vi "DAQ Thread_Gantner.vi"() -> ()   [LabVIEW 2016]
uses:
  HardWare/Gantner/HW_DevInfo.ctl
  HardWare/Gantner/HW_Module Info.ctl
  HardWare/Ctrls/HardWare Basic Info _ Channel.ctl
  HardWare/Ctrls/HardWare _ Channel Parameters.ctl
  Ctrls/Read and Write Ring.ctl
  HardWare/Gantner/DAQ FGV Operations.ctl
  Architecture/Queue Management/ARC_Queue Create_Single.vi
  Architecture/Queue Management/ARC_Queue Valid.vi
  Architecture/Queue Management/ARC_Queue Remove Element.vi
  Architecture/Queue Management/ARC_Queue Insert Element.vi
  Architecture/Queue Management/ARC_Queue Destroy_Single.vi
  <vilib>/Utility/error.llb/DialogType.ctl
panel:
  in  "daq?":bool
  in  "Parameter":cluster{"Q-Local":string, "Variant":variant}
  out "Error Report":string
  out "Current State":string
  in  "Exit Program":bool
  in  "TempVariable":T5
  # "/* -------- Notes for All Users -------- */\nRecommand : \n[1].Display Setting Resolution -> 1440x900\n[2].Read Arch Notes First.\n[3].Make A Call When You Are In Trouble.\n\nTeam Members:\nPansino Soft,Pansino SDMA\n\nCopyright@2013 Pansino.Beijing\n\nVersion Number: 2013"
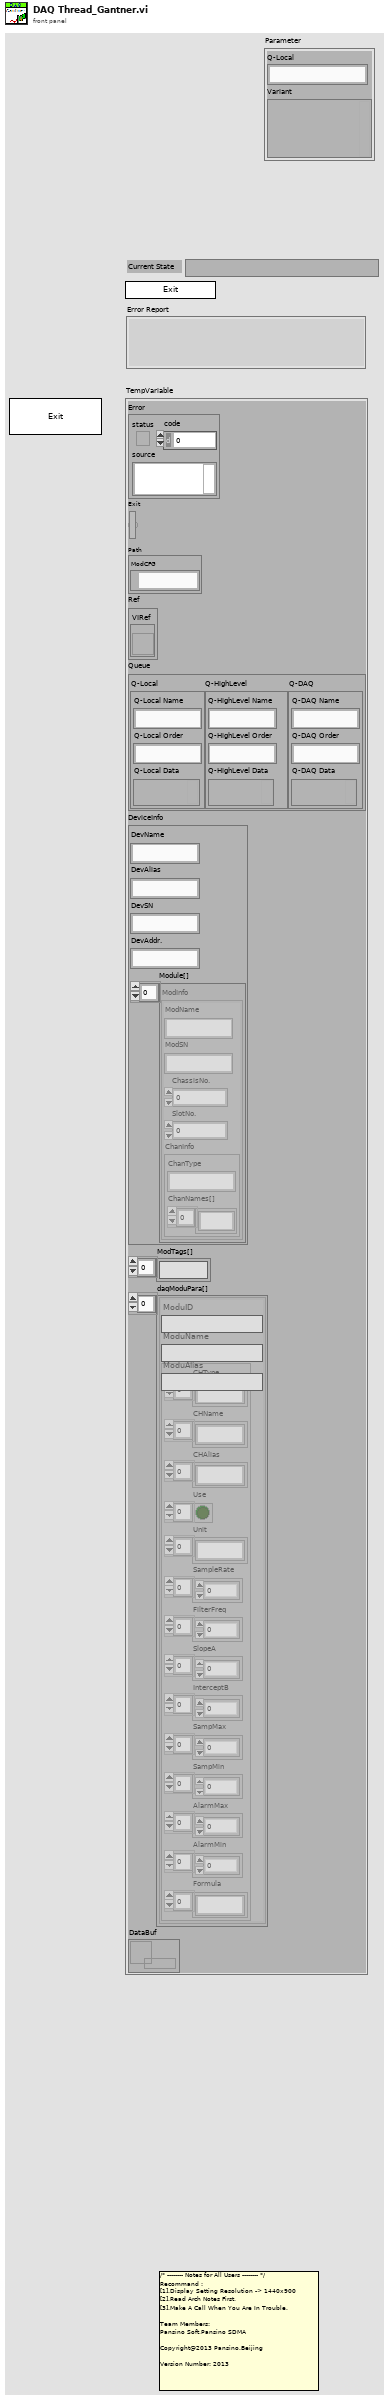
[diagram p1: front panel]
types:
  T1 = typedef "HW_DevInfo.ctl" = cluster{"DevName":string, "DevAlias":string, "DevSN":string, "DevAddr.":string, "Module[]":T2[]}
  T2 = typedef "HW_Module Info.ctl" = cluster{"ModName":string, "ModSN":string, "ChassisNo.":u32, "SlotNo.":u32, "ChanInfo":T3}
  T3 = typedef "HardWare Basic Info _ Channel.ctl" = cluster{"ChanType":string, "ChanNames[]":string[]}
  T4 = typedef "HardWare _ Channel Parameters.ctl" = cluster{"CHType":string[], "CHName":string[], "CHAlias":string[], "Use":bool[], "Unit":string[], "SampleRate":dbl[], "FilterFreq":dbl[], "SlopeA":dbl[], "InterceptB":dbl[], "SampMax":dbl[], "SampMin":dbl[], "AlarmMax":dbl[], "AlarmMin":dbl[], "Formula":string[]}
  T5 = cluster{"Error":errorcluster, "Exit":bool, "Path":cluster{"ModCFG":path}, "Ref":cluster{"VIRef":refnum<vi>}, "Queue":cluster{"Q-Local":cluster{"Q-Local Name":string, "Q-Local Order":string, "Q-Local Data":variant}, "Q-HighLevel":cluster{"Q-HighLevel Name":string, "Q-HighLevel Order":string, "Q-HighLevel Data":variant}, "Q-DAQ":cluster{"Q-DAQ Name":string, "Q-DAQ Order":string, "Q-DAQ Data":variant}}, "DeviceInfo":T1, "ModTags[]":string[], "daqModuPara[]":cluster{"ModuID":string, "ModuName":string, "ModuAlias":string, "ChanPara":T4}[], "DataBuf":refnum<queue>}
  T6 = cluster{"Q-Local Name":string, "DataBuf":refnum<queue>}
  T7 = typedef "DAQ FGV Operations.ctl" = enum16{"Search", "ReadCFG", "ReadVCH", "UpdateTempCFG", "DownloadCFG", "OpenCFG", "ImportPara", "Config", "Start", "Read", "Stop", "Clear"}
  T8 = typedef "Read and Write Ring.ctl" = enum16{"Read", "Write"}
  T9 = typedef "DialogType.ctl" = u16
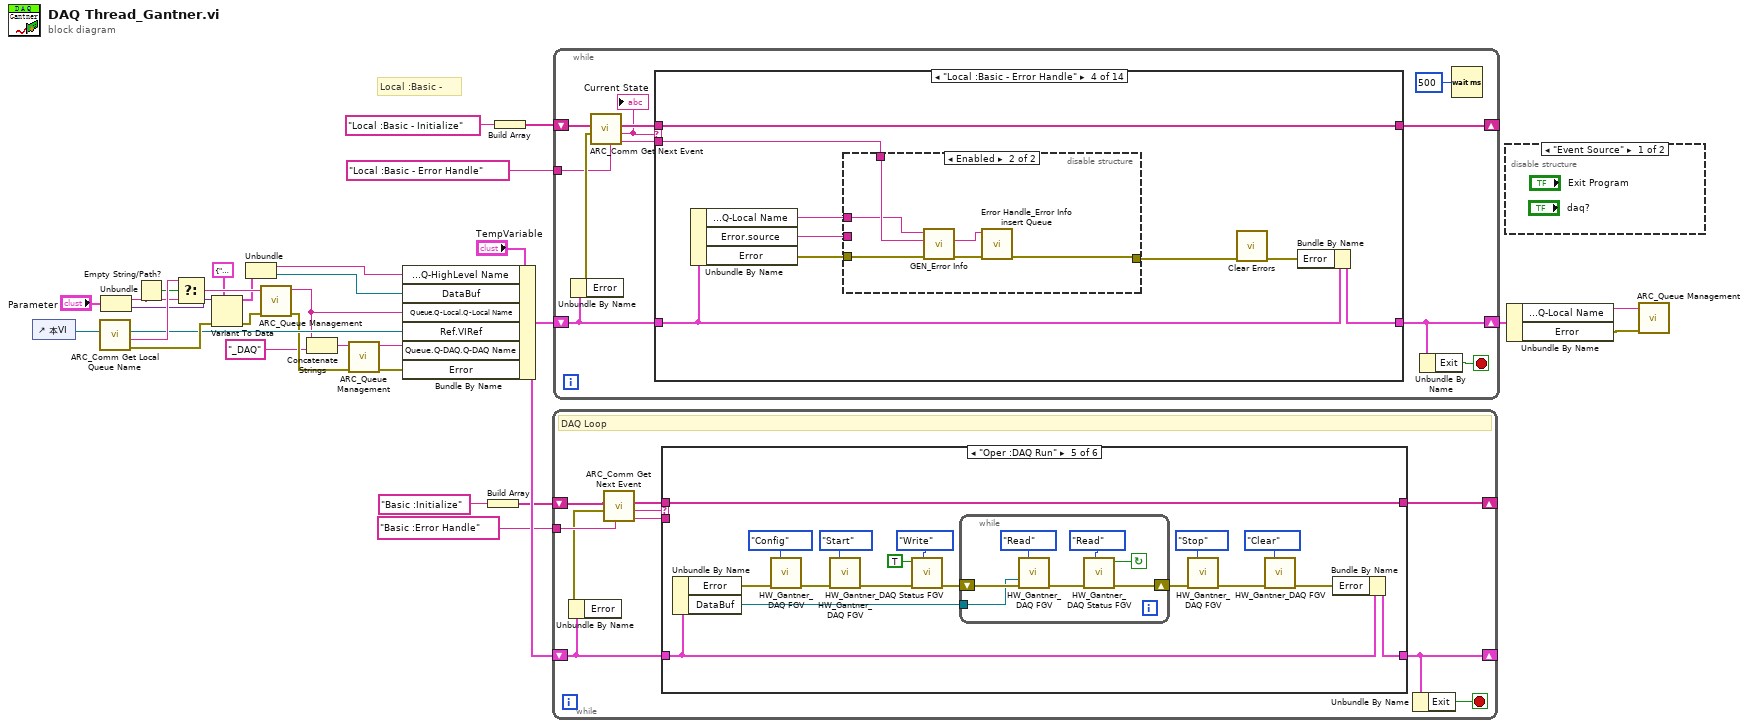
[diagram p0: block diagram]
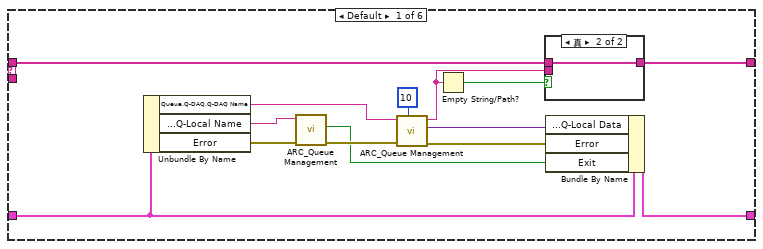
[diagram p2: hidden frame]
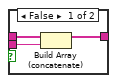
[diagram p3: hidden frame]
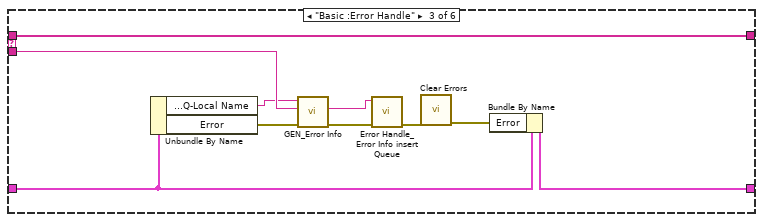
[diagram p5: hidden frame]
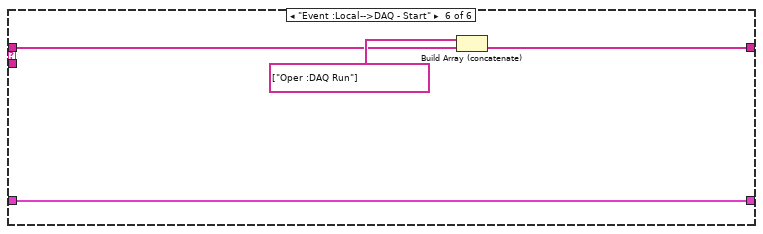
[diagram p7: hidden frame]
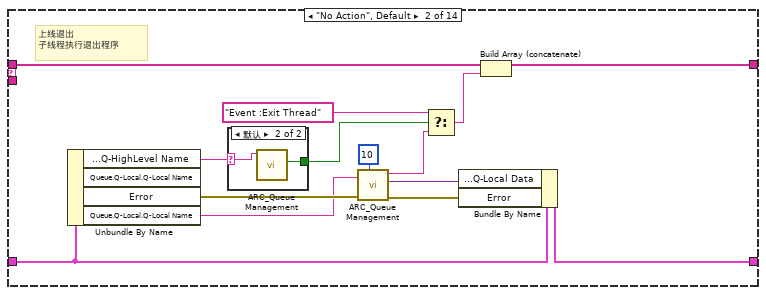
[diagram p10: hidden frame]
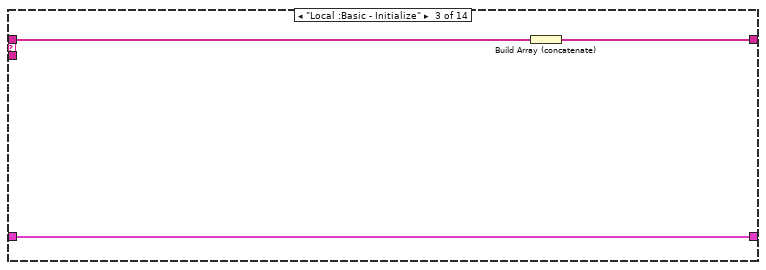
[diagram p12: hidden frame]
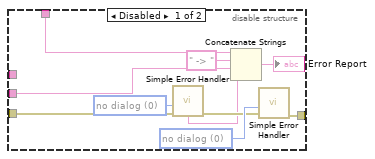
[diagram p13: hidden frame]
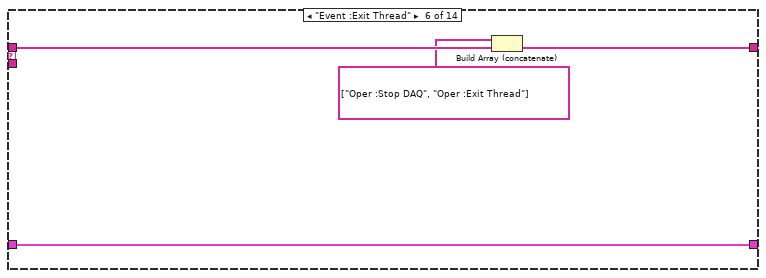
[diagram p15: hidden frame]
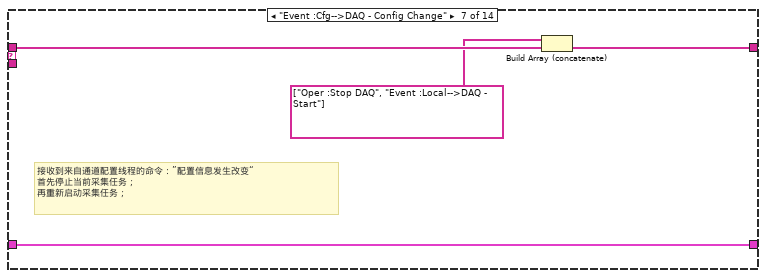
[diagram p16: hidden frame]
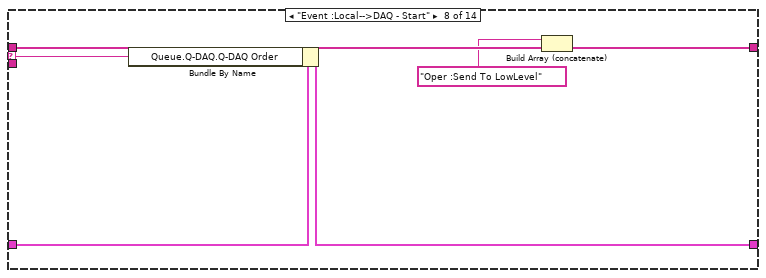
[diagram p17: hidden frame]
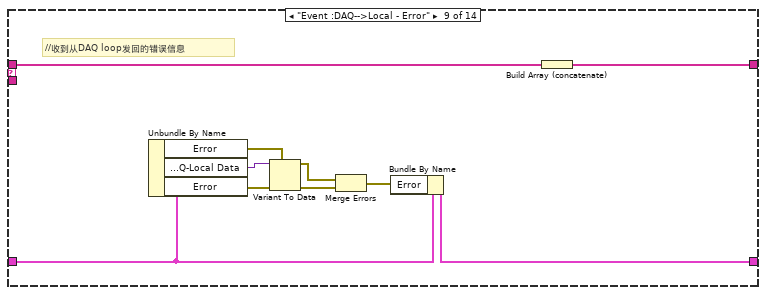
[diagram p18: hidden frame]
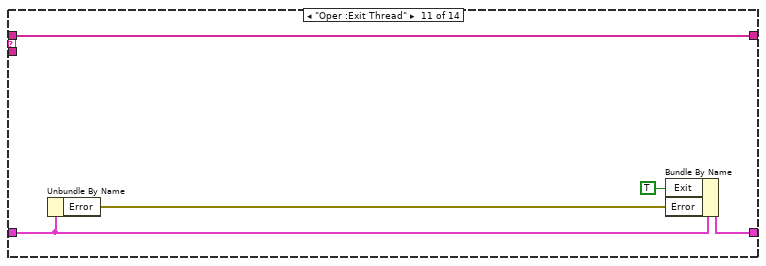
[diagram p20: hidden frame]
diagram:
  # "Local :Basic -"
  n1 = control-ref of="本VI"() -> (w19:refnum<vi>)
  n2 = call "ARC_Comm Get Local Queue Name.vi"("VI Ref"=w19) -> ("error out"=w20:errorcluster, "VI  Name"=w25:string, "VI Ref out"=w17:refnum<vi>)  [unwired: 8 in]
  n3 = Unbundle("Parameter") -> ("Q-Local"=w21:string, "Variant"=w24:variant)
  n4 = Empty String/Path?(string/path=w21) -> (empty?=w23:bool)
  n5 = Select(t=w25, s=w23, f=w21) -> (s? t:f=w7:string)
  n6 = Variant To Data(error in=w20, type=T6 {"Q-Local Name"="", "DataBuf"=refnum} ("output cluster"), Variant=w24) -> (data=w6:T6, error out=w18:errorcluster)
  n7 = Unbundle(w6) -> ("Q-Local Name"=w2:string, "DataBuf"=w1:refnum<queue>)
  n8 = call-poly "ARC_Queue Management.vi"("error in"=w18, "Queue Name"=w7) -> ("error out"=w15:errorcluster, "Queue Name dup"=w9:string)  [unwired: 7 in, 1 out]
  n9 = Concatenate Strings(w9, "_DAQ" ("字符串")) -> (w14:string)
  n10 = call-poly "ARC_Queue Management.vi"("error in"=w15, "Queue Name"=w14) -> ("error out"=w4:errorcluster, "Queue Name dup"=w5:string)  [unwired: 7 in, 1 out]
  n11 = Bundle By Name(cluster="TempVariable", "Queue.Q-HighLevel.Q-HighLevel Name"=w2, "DataBuf"=w1, "Queue.Q-Local.Q-Local Name"=w9, "Ref.VIRef"=w17, "Queue.Q-DAQ.Q-DAQ Name"=w5, "Error"=w4) -> (w16:T5)
  n12 = Build Array("Basic :Initialize") -> (w11:string[])
  n13 = Build Array("Local :Basic - Initialize") -> (w26:string[])
  n14 = while {
    shift-right: [w35] -> _
    shift-left: w11 -> [w41]
    tunnel: "Basic :Error Handle" ("Error Handle") -> [w39]
    shift-right: [w34] -> _
    shift-left: w16 -> [w36]
    stop <- w33 stop-if-true
    # "DAQ Loop"
    n15 = Unbundle By Name(w36) -> ("Error"=w38:errorcluster)
    n16 = call "ARC_Comm Get Next Event.vi"("Error Handle"=w39, "error in (no error)"=w38, "event queue in"=w41) -> ("prev event"=w32:string, "next event"=w37:string, "event queue out"=w40:string[])  [unwired: 3 in]
    n17 = case shown="\"Oper :DAQ Run\"" w37 {
      tunnel: w40 -> [w55 w60 w71 w72 w90 w99]
      tunnel: w36 -> [w50 w61 w70 w73 w88 w100]
      tunnel: [w51 w61 w69 w73 w89 w100] -> w34
      tunnel: [w45 w60 w71 w72 w90 w98] -> w35
      tunnel: w32 -> [_ _ w63 _ _ _]
      frame Default {
        n18 = Unbundle By Name(w50) -> ("Queue.Q-DAQ.Q-DAQ Name"=w46:string, "Queue.Q-Local.Q-Local Name"=w49:string, "Error"=w48:errorcluster)
        n19 = call-poly "ARC_Queue Management.vi"("error in (no error)"=w48, "Queue Name(unamed)"=w49) -> ("error out"=w47:errorcluster, "Not Exist?"=w42:bool)  [unwired: 7 in, 1 out]
        n20 = call-poly "ARC_Queue Management.vi"("Time out(-1)_queue out"=10, "error in (no error)"=w47, "Queue Name(unamed)"=w46) -> ("error out"=w52:errorcluster, "Data"=w53:variant, "Event"=w44:string)  [unwired: 5 in, 1 out]
        n21 = Empty String/Path?(string/path=w44) -> (empty?=w43:bool)
        n22 = case shown="真" w43 {
          tunnel: w55 -> [w58 w59]
          tunnel: [w57 w59] -> w45
          tunnel: w44 -> [w56 _]
          frame False {
            n23 = Build Array (concatenate)(w58, w56) -> (w57:string[])
          }
          frame True {
          }
        }
        n24 = Bundle By Name(cluster=w50, "Queue.Q-Local.Q-Local Data"=w53, "Error"=w52, "Exit"=w42) -> (w51:T5)
      }
      frame "Basic :Initialize" {
      }
      frame "Basic :Error Handle" {
        n25 = Unbundle By Name(w70) -> ("Queue.Q-Local.Q-Local Name"=w62:string, "Error"=w67:errorcluster)
        n26 = call "GEN_Error Info.vi"("error in"=w67, "Event name"=w63, "Thread name"=w62) -> ("error out"=w66:errorcluster, "Error Report"=w64:string)  [unwired: 7 in]
        n27 = call "Error Handle_Error Info insert Queue.vi"("error in"=w66, "error info in"=w64) -> ("error out"=w65:errorcluster)  [unwired: 9 in]
        n28 = call <vilib>:"Clear Errors.vi"("error in (no error)"=w65) -> ("error out"=w68:errorcluster)  [unwired: 5 in, 1 out]
        n29 = Bundle By Name(cluster=w70, "Error"=w68) -> (w69:T5)
      }
      frame "----------Operations-----------" {
      }
      frame "Oper :DAQ Run" {
        n30 = Unbundle By Name(w88) -> ("Error"=w87:errorcluster, "DataBuf"=w74:refnum<queue>)
        n31 = call "HW_Gantner_DAQ FGV.vi"("Oper."=DAQ_FGV_Operations."Config", "error in"=w87) -> ("error out"=w86:errorcluster)  [unwired: 7 in, 6 out]
        n32 = call "HW_Gantner_DAQ FGV.vi"("Oper."=DAQ_FGV_Operations."Start", "error in"=w86) -> ("error out"=w76:errorcluster)  [unwired: 7 in, 6 out]
        n33 = call "HW_Gantner_DAQ Status FGV.vi"("Oper"=Read_and_Write_Ring."Write", "error in"=w76, "DAQ Status in"=TRUE) -> ("error out"=w75:errorcluster)  [unwired: 7 in, 1 out]
        n34 = while {
          shift-right: [w92] -> w81
          shift-left: w75 -> [w97]
          tunnel: w74 -> [w91]
          stop <- w93 continue-if-true
          n35 = call "HW_Gantner_DAQ FGV.vi"("Oper."=DAQ_FGV_Operations."Read", "DataBuf"=w91, "error in"=w97) -> ("error out"=w94:errorcluster)  [unwired: 6 in, 6 out]
          n36 = call "HW_Gantner_DAQ Status FGV.vi"("Oper"=Read_and_Write_Ring."Read", "error in"=w94) -> ("error out"=w92:errorcluster, "DAQ Status out"=w93:bool)  [unwired: 8 in]
        }
        n37 = call "HW_Gantner_DAQ FGV.vi"("Oper."=DAQ_FGV_Operations."Stop", "error in"=w81) -> ("error out"=w80:errorcluster)  [unwired: 7 in, 6 out]
        n38 = call "HW_Gantner_DAQ FGV.vi"("Oper."=DAQ_FGV_Operations."Clear", "error in"=w80) -> ("error out"=w79:errorcluster)  [unwired: 7 in, 6 out]
        n39 = Bundle By Name(cluster=w88, "Error"=w79) -> (w89:T5)
      }
      frame "Event :Local-->DAQ - Start" {
        n40 = Build Array (concatenate)(string[] ["Oper :DAQ Run"] ("event queue out"), w99) -> (w98:string[])
      }
    }
    n41 = Unbundle By Name(w34) -> ("Exit"=w33:bool)
  }
  n42 = while {
    shift-right: [w107] -> w31
    shift-left: w16 -> [w109]
    shift-right: [w110] -> _
    shift-left: w26 -> [w112]
    tunnel: "Local :Basic - Error Handle" ("Error Handle") -> [w106]
    stop <- w102 stop-if-true
    n43 = Unbundle By Name(w109) -> ("Error"=w108:errorcluster)
    n44 = call "ARC_Comm Get Next Event.vi"("Error Handle"=w106, "error in (no error)"=w108, "event queue in"=w112) -> ("prev event"=w105:string, "next event"=w104:string, "event queue out"=w111:string[])  [unwired: 3 in]
    "Current State" <- w104
    n45 = case shown="\"Local :Basic - Error Handle\"" w104 {
      selector: w104 -> [_ _ _ _ _ _ _ w169 _ _ _ _ _ _]
      tunnel: w109 -> [w113 w128 w131 w140 w159 w163 w165 w173 w182 w185 w188 w197 w204 w220]
      tunnel: w111 -> [w114 w121 w133 w142 w160 w164 w168 w174 w184 w186 w191 w198 w207 w223]
      tunnel: [w114 w120 w132 w142 w160 w162 w167 w172 w183 w186 w191 w198 w207 w223] -> w110
      tunnel: [w113 w127 w131 w141 w159 w163 w165 w170 w178 w185 w189 w195 w203 w219] -> w107
      tunnel: w105 -> [_ _ _ w137 _ _ _ _ _ _ _ _ _ _]
      frame "----------Core Status----------" {
      }
      frame "No Action", Default {
        # "上线退出\n子线程执行退出程序"
        n46 = Unbundle By Name(w128) -> ("Queue.Q-HighLevel.Q-HighLevel Name"=w123:string, "Error"=w124:errorcluster, "Queue.Q-Local.Q-Local Name"=w122:string)  [unwired: 1 out]
        n47 = case shown="默认" w123 {
          selector: w123 -> [_ w129]
          tunnel: [_ w130] -> w115
          frame "" {
          }
          frame Default {
            n48 = call-poly "ARC_Queue Management.vi"("Queue Name(unamed)"=w129) -> ("Not Exist?"=w130:bool)  [unwired: 8 in, 2 out]
          }
        }
        n49 = call-poly "ARC_Queue Management.vi"("Time out(-1)_queue out"=10, "error in (no error)"=w124, "Queue Name(unamed)"=w122) -> ("error out"=w126:errorcluster, "Data"=w125:variant, "Event"=w117:string)  [unwired: 5 in, 1 out]
        n50 = Select(t="Event :Exit Thread" ("Event"), s=w115, f=w117) -> (s? t:f=w116:string)
        n51 = Bundle By Name(cluster=w128, "Queue.Q-Local.Q-Local Data"=w125, "Error"=w126) -> (w127:T5)
        n52 = Build Array (concatenate)(w121, w116) -> (w120:string[])
      }
      frame "Local :Basic - Initialize" {
        n53 = Build Array (concatenate)(w133) -> (w132:string[])
      }
      frame "Local :Basic - Error Handle" {
        n54 = Unbundle By Name(w140) -> ("Queue.Q-Local.Q-Local Name"=w134:string, "Error.source"=w136:string, "Error"=w138:errorcluster)
        n55 = disable-structure shown="Enabled" {
          disable-tunnel: w138 -> [w152 w156]
          disable-tunnel: w137 -> [w151 w154]
          disable-tunnel: w136 -> [w150 _]
          disable-tunnel: [w149 w155] -> w135
          disable-tunnel: w134 -> [_ w153]
          frame Disabled {
            w146 = T9 0 items=["no dialog", "OK message", "continue or stop message", "OK message + warnings", "continue/stop + warnings"] ("type of dialog (OK msg:1)")
            w148 = T9 0 items=["no dialog", "OK message", "continue or stop message", "OK message + warnings", "continue/stop + warnings"] ("type of dialog (OK msg:1)")
            n56 = call <vilib>:"Simple Error Handler.vi"("type of dialog (OK msg:1)"=w146, "error in (no error)"=w152) -> ("error out"=w147:errorcluster, "message"=w144:string)  [unwired: 3 in, 3 out]
            n57 = Concatenate Strings(w151, " -> " ("字符串"), w150, w144) -> (→"Error Report":string)
            n58 = call <vilib>:"Simple Error Handler.vi"("type of dialog (OK msg:1)"=w148, "error in (no error)"=w147) -> ("error out"=w149:errorcluster)  [unwired: 3 in, 4 out]
          }
          frame Enabled {
            n59 = call "GEN_Error Info.vi"("error in"=w156, "Event name"=w154, "Thread name"=w153) -> ("error out"=w157:errorcluster, "Error Report"=w158:string)  [unwired: 7 in]
            n60 = call "Error Handle_Error Info insert Queue.vi"("error in"=w157, "error info in"=w158) -> ("error out"=w155:errorcluster)  [unwired: 9 in]
          }
        }
        n61 = call <vilib>:"Clear Errors.vi"("error in (no error)"=w135) -> ("error out"=w139:errorcluster)  [unwired: 5 in, 1 out]
        n62 = Bundle By Name(cluster=w140, "Error"=w139) -> (w141:T5)
      }
      frame "----------event----------" {
      }
      frame "Event :Exit Thread" {
        n63 = Build Array (concatenate)(string[] ["Oper :Stop DAQ", "Oper :Exit Thread"] ("数组"), w164) -> (w162:string[])
      }
      frame "Event :Cfg-->DAQ - Config Change" {
        # "接收到来自通道配置线程的命令：”配置信息发生改变“\n首先停止当前采集任务；\n再重新启动采集任务；"
        n64 = Build Array (concatenate)(string[] ["Oper :Stop DAQ", "Event :Local-->DAQ - Start"] ("event queue out"), w168) -> (w167:string[])
      }
      frame "Event :Local-->DAQ - Start" {
        n65 = Bundle By Name(cluster=w173, "Queue.Q-DAQ.Q-DAQ Order"=w169) -> (w170:T5)
        n66 = Build Array (concatenate)("Oper :Send To LowLevel" ("Error Handle"), w174) -> (w172:string[])
      }
      frame "Event :DAQ-->Local - Error" {
        # "//收到从DAQ loop发回的错误信息"
        n67 = Unbundle By Name(w182) -> ("Error"=w179:errorcluster, "Queue.Q-Local.Q-Local Data"=w180:variant, "Error"=w181:errorcluster)
        n68 = Variant To Data(error in=w181, type=w179, Variant=w180) -> (data=w175:errorcluster, error out=w177:errorcluster)
        n69 = Merge Errors(w175, w177) -> (w176:errorcluster)
        n70 = Bundle By Name(cluster=w182, "Error"=w176) -> (w178:T5)
        n71 = Build Array (concatenate)(w184) -> (w183:string[])
      }
      frame "----------Operation----------" {
      }
      frame "Oper :Exit Thread" {
        n72 = Unbundle By Name(w188) -> ("Error"=w190:errorcluster)
        n73 = Bundle By Name(cluster=w188, "Exit"=TRUE, "Error"=w190) -> (w189:T5)
      }
      frame "Oper :Stop DAQ" {
        # "状态变量写入停止采集"
        n74 = Unbundle By Name(w197) -> ("Error"=w196:errorcluster)
        n75 = call "HW_Gantner_DAQ Status FGV.vi"("Oper"=Read_and_Write_Ring."Write", "error in"=w196, "DAQ Status in"=FALSE) -> ("error out"=w194:errorcluster)  [unwired: 7 in, 1 out]
        n76 = Bundle By Name(cluster=w197, "Error"=w194) -> (w195:T5)
      }
      frame "Oper :Send To HighLevel" {
        n77 = Unbundle By Name(w204) -> ("Queue.Q-HighLevel.Q-HighLevel Name"=w206:string, "Queue.Q-HighLevel.Q-HighLevel Order"=w201:string, "Queue.Q-HighLevel.Q-HighLevel Data"=w200:variant, "Error"=w205:errorcluster)
        n78 = call-poly "ARC_Queue Management.vi"("Queue Name(unamed)"=w206) -> ("Not Exist?"=w202:bool)  [unwired: 8 in, 2 out]
        n79 = case shown="假" w202 {
          tunnel: w205 -> [w213 w214]
          tunnel: w206 -> [w211 _]
          tunnel: w201 -> [w209 _]
          tunnel: w200 -> [w210 _]
          tunnel: [w208 w214] -> w199
          frame False {
            n80 = call-poly "ARC_Queue Management.vi"("Time out(-1)_queue in"=50, "error in (no error)"=w213, "Data"=w210, "Event"=w209, "Queue Name(unamed)"=w211) -> ("error out"=w208:errorcluster)  [unwired: 5 in, 1 out]
          }
          frame True {
          }
        }
        n81 = Bundle By Name(cluster=w204, "Error"=w199) -> (w203:T5)
      }
      frame "Oper :Send To LowLevel" {
        n82 = Unbundle By Name(w220) -> ("Queue.Q-DAQ.Q-DAQ Name"=w222:string, "Queue.Q-DAQ.Q-DAQ Order"=w217:string, "Queue.Q-DAQ.Q-DAQ Data"=w216:variant, "Error"=w221:errorcluster)
        n83 = call-poly "ARC_Queue Management.vi"("Queue Name(unamed)"=w222) -> ("Not Exist?"=w218:bool)  [unwired: 8 in, 2 out]
        n84 = case shown="假" w218 {
          tunnel: w221 -> [w229 w230]
          tunnel: w222 -> [w227 _]
          tunnel: w217 -> [w225 _]
          tunnel: w216 -> [w226 _]
          tunnel: [w224 w230] -> w215
          frame False {
            n85 = call-poly "ARC_Queue Management.vi"("Time out(-1)_queue in"=50, "error in (no error)"=w229, "Data"=w226, "Event"=w225, "Queue Name(unamed)"=w227) -> ("error out"=w224:errorcluster)  [unwired: 5 in, 1 out]
          }
          frame True {
          }
        }
        n86 = Bundle By Name(cluster=w220, "Error"=w215) -> (w219:T5)
      }
    }
    n87 = Unbundle By Name(w107) -> ("Exit"=w102:bool)
    n88 = Wait (ms)(milliseconds to wait=u32 500) -> ()  [unwired: 1 out]
  }
  n89 = disable-structure shown="\"Event Source\"" {
    frame condition #0 (active) {
    }
    frame condition #1 {
    }
  }
  n90 = Unbundle By Name(w31) -> ("Queue.Q-Local.Q-Local Name"=w8:string, "Error"=w30:errorcluster)
  n91 = call-poly "ARC_Queue Management.vi"("error in (no error)"=w30, "Queue Name(unamed)"=w8) -> ()  [unwired: 7 in, 3 out]
